vi "lowpass filter.vi"(1 "Integration Period (s)":dbl caption="Sampling Freq" format="%.2f", 2 "initialize filters":bool, 3 "Sampling Freq":dbl format="%.2f", 5 "INPUT":T2 {"Array" format="%.2f"; "Ch 2 Mult" format="%.2f"; "Ch 1 Mult" format="%.2f"; "LOCK-IN Freq" format="%.2f"; "LOCK-IN Phase" format="%.2f"; "Time Constant (sec)" format="%.2f"; "Low-pass filter slope" format="%.2f"; "Time" format="%.2f"; "Noise Amplitude" format="%.2f"; "Phase Angle" format="%.2f"; "Frequency" format="%.2f"; "Amplitude" format="%.2f"}) -> (0 "OUTPUT":T1 {"Input Signal" format="%.2f"; "X-Y Data"."Current Queue" format="%.2f"; "X-Y Data"."Current Queue" format="%.2f"; "Phase Difference" format="%.2f"; "Input Signal Amp" format="%.2f"; "Ch 2 Output" format="%.2f"; "Ch 1 Output" format="%.2f"})   [LabVIEW 2013]
doc: "Puts the Lock-In output through a low-pass filter in order to eliminate oscillations in the output."
uses:
  <vilib>/ptbypt/NI_PtbyPt.lvlib
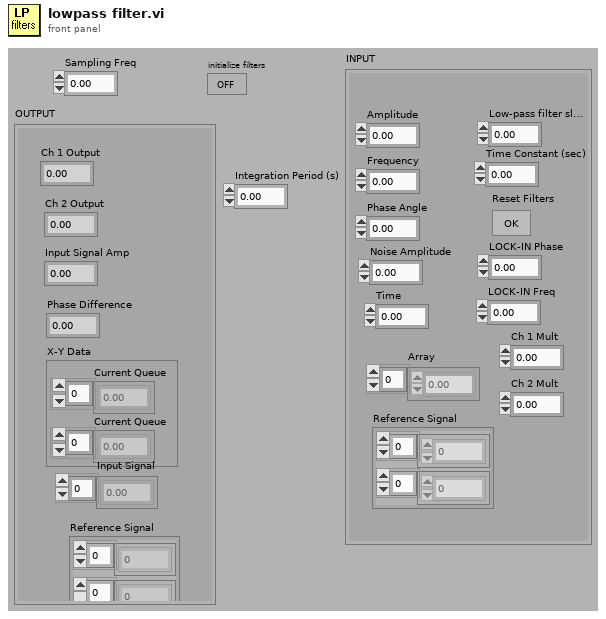
[diagram p1: front panel]
types:
  T1 = cluster{"Ch 1 Output":dbl, "Ch 2 Output":dbl, "Input Signal Amp":dbl, "Phase Difference":dbl, "X-Y Data":cluster{"Current Queue":dbl[], "Current Queue":dbl[]}, "Input Signal":dbl[], "Reference Signal":cluster{dbl[], dbl[]}}
  T2 = cluster{"Amplitude":dbl, "Frequency":dbl, "Phase Angle":dbl, "Noise Amplitude":dbl, "Time":dbl, "Low-pass filter slope":dbl, "Time Constant (sec)":dbl, "Reset Filters":bool, "LOCK-IN Phase":dbl, "LOCK-IN Freq":dbl, "Array":dbl[], "Ch 1 Mult":dbl, "Ch 2 Mult":dbl, "Reference Signal":cluster{dbl[], dbl[]}}
  T3 = enum16{"Lowpass", "Highpass", "Bandpass", "Bandstop"}
  T4 = cluster{"Current Queue":dbl[], "Current Queue":dbl[]}
  T5 = cluster{"Filtered x":dbl, "Filtered x":dbl, dbl, dbl, cluster{"Current Queue":dbl[], "Current Queue":dbl[]}, "Array":dbl[], "Reference Signal":cluster{dbl[], dbl[]}}
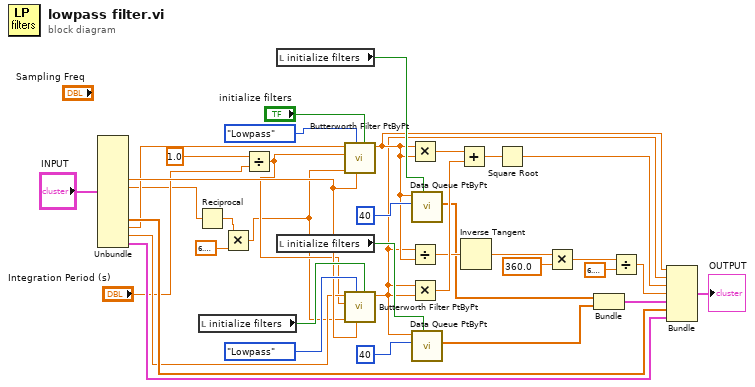
[diagram p0: block diagram]
diagram:
  n1 = Unbundle("INPUT") -> ("Low-pass filter slope"=w19:dbl, "Time Constant (sec)"=w4:dbl, "Array"=w14:dbl[], "Ch 1 Mult"=w13:dbl, "Ch 2 Mult"=w12:dbl, "Reference Signal"=w11:cluster{dbl[], dbl[]})  [unwired: 8 out]
  n2 = Reciprocal(x=w4) -> (1/x=w2:dbl)
  n3 = local read "initialize filters"() -> (w23:bool)
  n4 = Multiply(x=w2, y=6.283185307179586) -> (x*y=w1:dbl)
  n5 = Divide(x=1.0, y="Integration Period (s)") -> (x/y=w5:dbl)
  n6 = local read "initialize filters"() -> (w21:bool)
  n7 = local read "initialize filters"() -> (w22:bool)
  n8 = call <vilib>:"Butterworth Filter PtByPt.vi"("initialize"="initialize filters", "order"=w19, "filter type"=T3."Lowpass", "low cutoff freq: fl"=w1, "sampling freq: fs"=w5, "x"=w13) -> ("Filtered x"=w9:dbl)  [unwired: 3 in, 1 out]
  n9 = call <vilib>:"Butterworth Filter PtByPt.vi"("initialize"=w23, "order"=w19, "filter type"=T3."Lowpass", "low cutoff freq: fl"=w1, "sampling freq: fs"=w5, "x"=w12) -> ("Filtered x"=w8:dbl)  [unwired: 3 in, 1 out]
  n10 = Multiply(x=w9, y=w9) -> (x*y=w35:dbl)
  n11 = Divide(x=w8, y=w9) -> (x/y=w32:dbl)
  n12 = Multiply(x=w8, y=w8) -> (x*y=w34:dbl)
  n13 = call <vilib>:"Data Queue PtByPt.vi"("initialize"=w21, "sample length"=40, "input data point"=w9) -> ("Current Queue"=w25:dbl[])  [unwired: 4 in, 4 out]
  n14 = call <vilib>:"Data Queue PtByPt.vi"("initialize"=w22, "sample length"=40, "input data point"=w8) -> ("Current Queue"=w24:dbl[])  [unwired: 4 in, 4 out]
  n15 = Add(x=w35, y=w34) -> (x+y=w33:dbl)
  n16 = Inverse Tangent(1:w32) -> (0:w31:dbl)
  n17 = Square Root(x=w33) -> (sqrt(x)=w16:dbl)
  n18 = Multiply(x=w31, y=360.0) -> (x*y=w28:dbl)
  n19 = Bundle("Current Queue"=w25, "Current Queue"=w24) -> (w17:T4)  [unwired: 1 in]
  n20 = Divide(x=w28, y=6.283185307179586) -> (x/y=w15:dbl)
  n21 = Bundle("Filtered x"=w9, "Filtered x"=w8, w16, w15, w17, "Array"=w14, "Reference Signal"=w11) -> (→"OUTPUT":T5)  [unwired: 1 in]
